vi "Main VI Stand-Alone Prevent Trip.vi"() -> ()   [LabVIEW 2020]
panel:
  in  "stop":bool
  out "Power Supply Trip":bool
  in  "Power Supply \nAddress":refnum<visa-resource-name>
  in  "Barcodes in":string[](array[string])
  in  "Barcodes in 2":string[](array[string])
  in  "Barcodes in 3":string[](array[string])
  in  "Barcodes in 4":string[](array[string])
  out "Elapsed Time (s)":dbl
  in  "Start":bool
  out "Test Is Running (Red)\nTest Is Stopped (Green)":bool
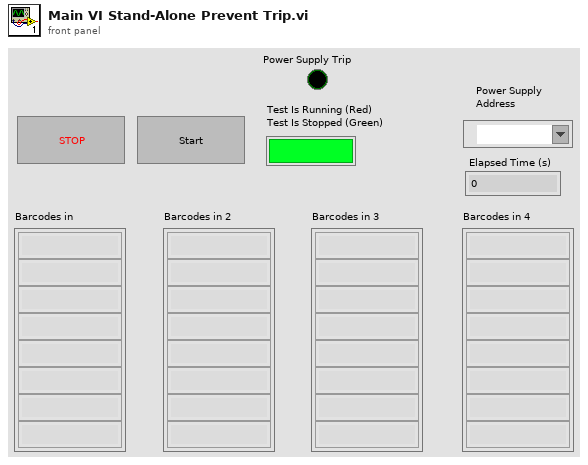
[diagram p1: front panel]
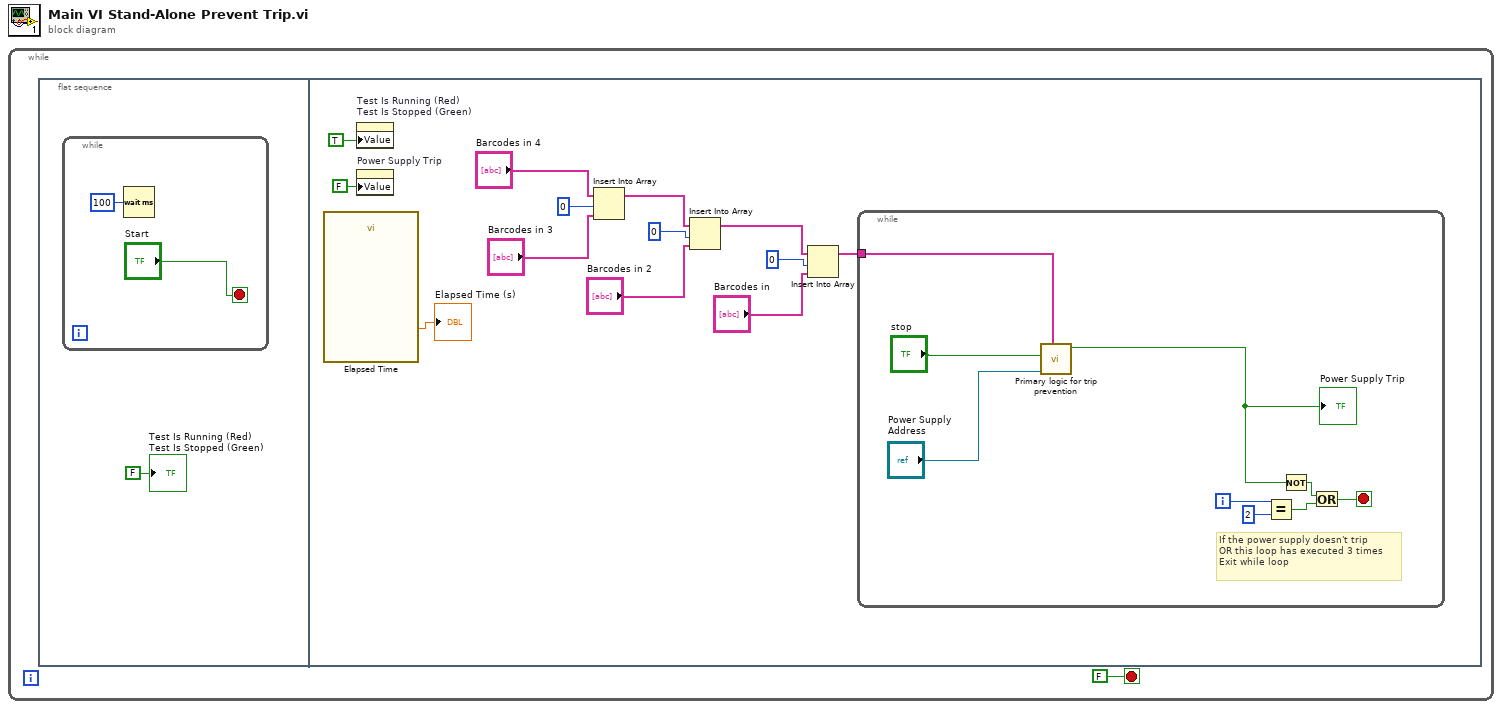
[diagram p0: block diagram]
diagram:
  n1 = while {
    stop <- FALSE stop-if-true
    n2 = flat-sequence {
      frame #0 {
        n3 = while {
          stop <- "Start" stop-if-true
          n4 = Wait (ms)(milliseconds to wait=u32 100) -> ()  [unwired: 1 out]
        }
        "Test Is Running (Red)\nTest Is Stopped (Green)" <- FALSE ("Start LED")
      }
      frame #1 {
        n5 = call "Elapsed Time"() -> ("Elapsed Time (s)"=→"Elapsed Time (s)":dbl)  [unwired: 12 in, 7 out]
        n6 = property on="Test Is Running (Red)\nTest Is Stopped (Green)" class="Bool (strict)"("Value"=TRUE) -> ()  [unwired: 2 in, 2 out]
        n7 = property on="Power Supply Trip" class="Bool (strict)"("Value"=FALSE ("Power Supply Trip")) -> ()  [unwired: 2 in, 2 out]
        n8 = Insert Into Array(array="Barcodes in 4", index=0, new element="Barcodes in 3") -> (w11:string[])
        n9 = Insert Into Array(array=w11, index=0, new element="Barcodes in 2") -> (w7:string[])
        n10 = Insert Into Array(array=w7, index=0, new element="Barcodes in") -> (w6:string[])
        n11 = while {
          tunnel: w6 -> [w18]
          i -> [w25]
          stop <- w22 stop-if-true
          # "If the power supply doesn't trip\nOR this loop has executed 3 times Exit while loop"
          n12 = call "Primary logic for trip prevention.vi"("Barcodes in"=w18, "VISA Refnum in"="Power Supply \nAddress", "Stop Program"="stop") -> ("Power Supply Trip"=w19:bool)  [unwired: 8 in]
          "Power Supply Trip" <- w19
          n13 = Equal?(x=w25, y=2) -> (x = y?=w23:bool)
          n14 = Not(x=w19) -> (.not. x?=w26:bool)
          n15 = Or(x=w26, y=w23) -> (x .or. y?=w22:bool)
        }
      }
    }
  }
